vi "PAS_CFG.vi"(0 "TCP Network Connection in":refnum<k5>, 1 "INIT":bool, 2 "pAs_REG":u32=100, 5 "error in (no error)":errorcluster) -> (14 "TCP Network Connection out":refnum<k5>, 15 "pAs_STATUS":u8[](array[numeric]), 17 "PAM_INIT":u8[](array[numeric]), 19 "error out":errorcluster)   [LabVIEW 2019]
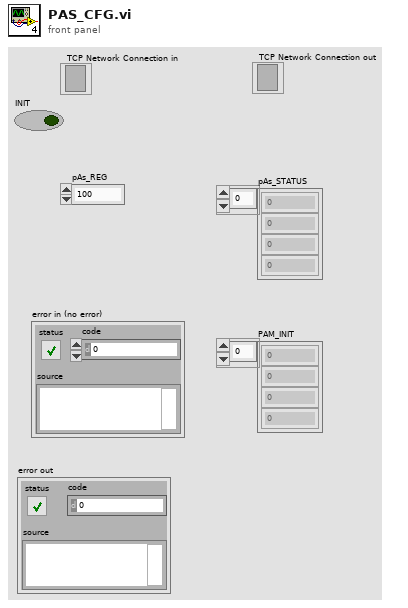
[diagram p1: front panel]
types:
  T1 = enum16{"big-endian, network order", "native, host order", "little-endian"}
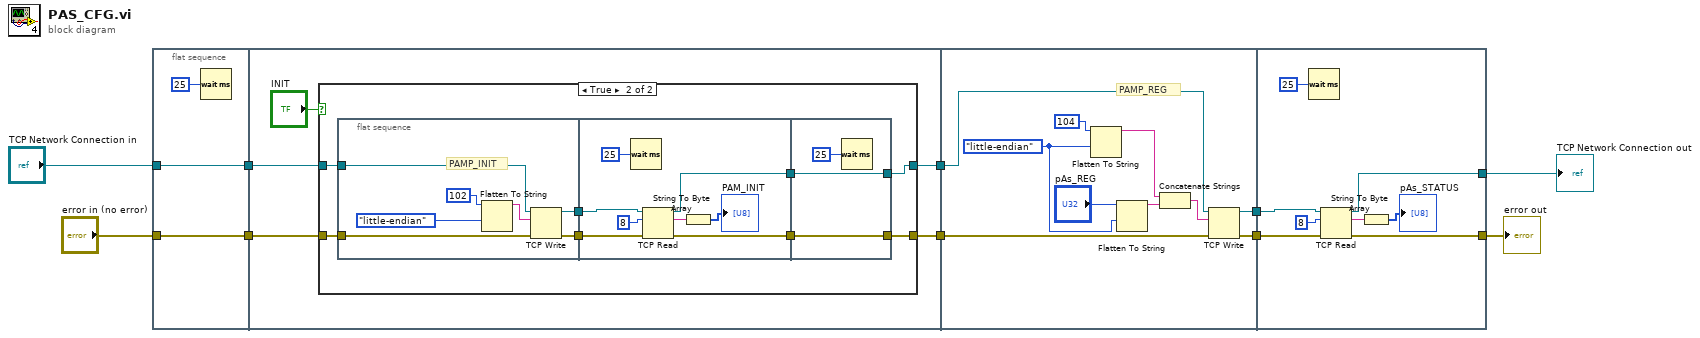
[diagram p0: block diagram]
diagram:
  n1 = flat-sequence {
    tunnel: [w12] -> w4
    tunnel: [w13] -> w2
    tunnel: "error in (no error)" -> [w13]
    tunnel: "TCP Network Connection in" -> [w12]
    tunnel: w4 -> [w18]
    tunnel: [w16] -> w3
    tunnel: w2 -> [w17]
    tunnel: [w15] -> w1
    tunnel: w3 -> [w56]
    tunnel: [w54] -> w6
    tunnel: [w53] -> w5
    tunnel: w1 -> [w55]
    tunnel: [w61] -> w8
    tunnel: [w62] -> w7
    tunnel: w6 -> [w64]
    tunnel: w5 -> [w63]
    frame #0 {
      n2 = Wait (ms)(milliseconds to wait=u32 25) -> ()  [unwired: 1 out]
    }
    frame #1 {
      n3 = case shown="True" "INIT" {
        tunnel: w18 -> [w20 w26]
        tunnel: w17 -> [w19 w25]
        tunnel: [w20 w24] -> w16
        tunnel: [w19 w23] -> w15
        frame False {
        }
        frame True {
          n4 = flat-sequence {
            tunnel: [w33] -> w28
            tunnel: [w32] -> w27
            tunnel: w26 -> [w35]
            tunnel: w25 -> [w34]
            tunnel: w28 -> [w43]
            tunnel: w27 -> [w42]
            tunnel: [w41] -> w22
            tunnel: [w40] -> w21
            tunnel: [w45] -> w23
            tunnel: [w46] -> w24
            tunnel: w22 -> [w46]
            tunnel: w21 -> [w45]
            frame #0 {
              # "PAMP_INIT"
              n5 = Flatten To String(anything=u32 102 ("element"), byte order (0:big-endian, network order)=T1."little-endian") -> (data string=w29:string)  [unwired: 2 in, 2 out]
              n6 = TCP Write(connection ID=w35, data in=w29, error in (no error)=w34) -> (connection ID out=w33:refnum<k5>, error out=w32:errorcluster)  [unwired: 1 in, 1 out]
            }
            frame #1 {
              n7 = Wait (ms)(milliseconds to wait=u32 25) -> ()  [unwired: 1 out]
              n8 = TCP Read(connection ID=w43, bytes to read=8, error in (no error)=w42) -> (connection ID out=w41:refnum<k5>, data out=w37:string, error out=w40:errorcluster)  [unwired: 2 in]
              n9 = String To Byte Array(string=w37) -> (unsigned byte array=→"PAM_INIT":u8[])
            }
            frame #2 {
              n10 = Wait (ms)(milliseconds to wait=u32 25) -> ()  [unwired: 1 out]
            }
          }
        }
      }
    }
    frame #2 {
      w51 = T1."little-endian" ("byte order (0:big-endian, network order)")
      # "PAMP_REG"
      n11 = Flatten To String(anything=u32 104 ("element"), byte order (0:big-endian, network order)=w51) -> (data string=w49:string)  [unwired: 2 in, 2 out]
      n12 = Flatten To String(anything="pAs_REG", byte order (0:big-endian, network order)=w51) -> (data string=w52:string)  [unwired: 2 in, 2 out]
      n13 = Concatenate Strings(w49, w52) -> (w48:string)
      n14 = TCP Write(connection ID=w56, data in=w48, error in (no error)=w55) -> (connection ID out=w54:refnum<k5>, error out=w53:errorcluster)  [unwired: 1 in, 1 out]
    }
    frame #3 {
      n15 = Wait (ms)(milliseconds to wait=u32 25) -> ()  [unwired: 1 out]
      n16 = TCP Read(connection ID=w64, bytes to read=8, error in (no error)=w63) -> (connection ID out=w62:refnum<k5>, data out=w58:string, error out=w61:errorcluster)  [unwired: 2 in]
      n17 = String To Byte Array(string=w58) -> (unsigned byte array=→"pAs_STATUS":u8[])
    }
  }
  "error out" <- w8
  "TCP Network Connection out" <- w7
